vi "GetSerializableClassHeader.vi"(8 "error in (no error)":errorcluster, 10 "StructuredData":variant, 11 "BlueSerializer in":refnum<class "BlueSerializer.lvclass">) -> (0 "error out":errorcluster, 1 "header found?":bool, 2 "SerializedClassHeader (child,parent)":T1[](array[typedef]), 3 "BlueSerializer out":refnum<class "BlueSerializer.lvclass">)   [LabVIEW 2020, in "BlueSerialization.lvlib" / "BlueSerializer.lvclass"]
uses:
  BlueSerializer.lvclass
  ClassHeader.ctl
  <vilib>/Utility/EditLVLibs/LibVersion.ctl
  BlueSerializableClassName.vi
  <vilib>/Utility/error.llb/Error Cluster From Error Code.vi
  StringVersionToLibraryVersion.vi
  <vilib>/Utility/LVClass/Get LV Class Name.vi
  BlueSerializable/BlueSerializable.lvclass
  <vilib>/Utility/EditLVLibs/Edit LVLibs.lvlib
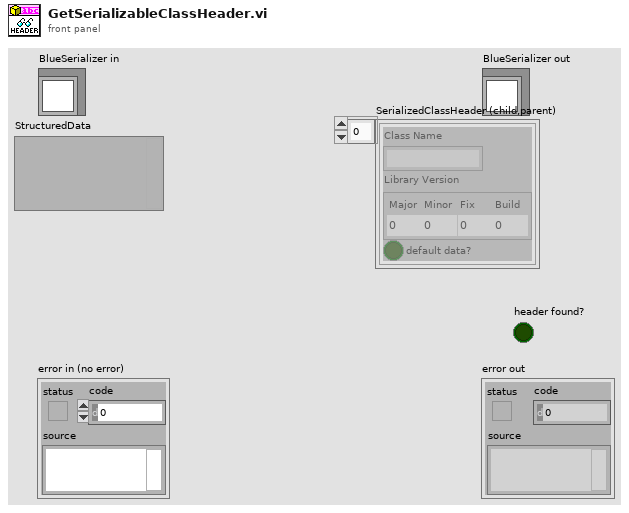
[diagram p1: front panel]
types:
  T1 = typedef "BlueSerialization.lvlib/BlueSerializer.lvclass/ClassHeader.ctl" = cluster{"Class Name":string, "Library Version":T2, "default data?":bool}
  T2 = typedef "Edit LVLibs.lvlib/LibVersion.ctl" = cluster{"Major":u16, "Minor":u16, "Fix":u16, "Build":u16}
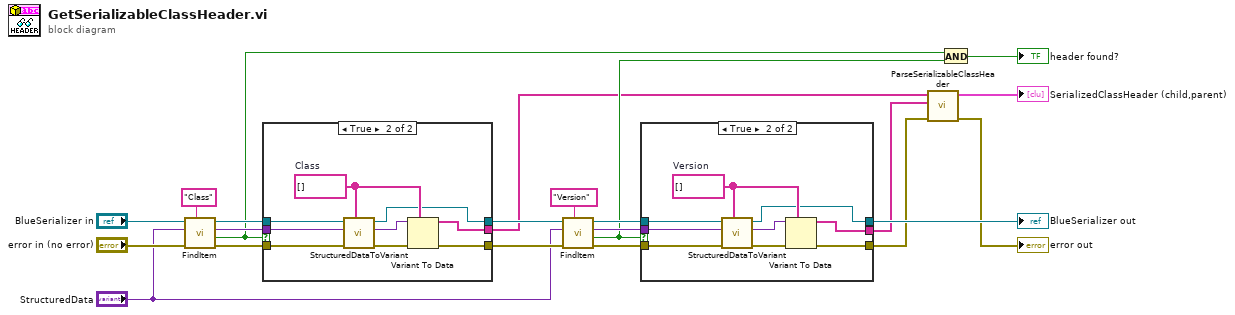
[diagram p0: block diagram]
diagram:
  n1 = call-dynamic "FindItem.vi"("Item Name"="Class", "error in (no error)"="error in (no error)", "StructuredDataContainer"="StructuredData", "BlueSerializer in"="BlueSerializer in") -> ("error out"=w17:errorcluster, "Found?"=w7:bool, "StructuredDataItem"=w18:variant, "BlueSerializer out"=w19:refnum<class "BlueSerializer.lvclass">)  [unwired: 4 in]
  n2 = case shown="True" w7 {
    tunnel: w19 -> [w23 w30]
    tunnel: w18 -> [_ w29]
    tunnel: w17 -> [w24 w28]
    tunnel: [_ w27] -> w4
    tunnel: [w24 w26] -> w12
    tunnel: [w23 w25] -> w11
    frame False {
    }
    frame True {
      w31 = string[] []  # Class
      n3 = call-dynamic "StructuredDataToVariant.vi"("Data Type"=w31, "error in (no error)"=w28, "StructuredData"=w29, "BlueSerializer in"=w30) -> ("error out"=w32:errorcluster, "Variant"=w33:variant, "BlueSerializer out"=w25:refnum<class "BlueSerializer.lvclass">)  [unwired: 5 in]
      n4 = Variant To Data(error in=w32, type=w31, Variant=w33) -> (data=w27:string[], error out=w26:errorcluster)
    }
  }
  n5 = call-dynamic "FindItem.vi"("Item Name"="Version", "error in (no error)"=w12, "StructuredDataContainer"="StructuredData", "BlueSerializer in"=w11) -> ("error out"=w16:errorcluster, "Found?"=w8:bool, "StructuredDataItem"=w15:variant, "BlueSerializer out"=w14:refnum<class "BlueSerializer.lvclass">)  [unwired: 4 in]
  n6 = case shown="True" w8 {
    tunnel: w14 -> [w34 w41]
    tunnel: w15 -> [_ w40]
    tunnel: w16 -> [w35 w39]
    tunnel: [_ w38] -> w5
    tunnel: [w35 w37] -> w3
    tunnel: [w34 w36] -> w10
    frame False {
    }
    frame True {
      w42 = string[] []  # Version
      n7 = call-dynamic "StructuredDataToVariant.vi"("Data Type"=w42, "error in (no error)"=w39, "StructuredData"=w40, "BlueSerializer in"=w41) -> ("error out"=w43:errorcluster, "Variant"=w44:variant, "BlueSerializer out"=w36:refnum<class "BlueSerializer.lvclass">)  [unwired: 5 in]
      n8 = Variant To Data(error in=w43, type=w42, Variant=w44) -> (data=w38:string[], error out=w37:errorcluster)
    }
  }
  "BlueSerializer out" <- w10
  n9 = call "ParseSerializableClassHeader.vi"("error in (no error)"=w3, "Version"=w5, "Class"=w4) -> ("error out"=→"error out":errorcluster, "SerializedClassHeader (child,parent)"=→"SerializedClassHeader (child,parent)":T1[])  [unwired: 7 in]
  n10 = And(x=w7, y=w8) -> (x .and. y?=→"header found?":bool)
